vi "OnFrameAvailable_Event_Callback.vi"(4 "User Parameter":T1, 5 "Event Data":cluster{"sender":refnum<k24>, "e":refnum<k24>}, 6 "Control Ref":refnum<k24>, 7 "Event Common Data":T2) -> ()   [LabVIEW 2018]
uses:
  C:/Program Files/Spiricon/BeamSquared/M2.Automation.dll
  M2.Automation.dll
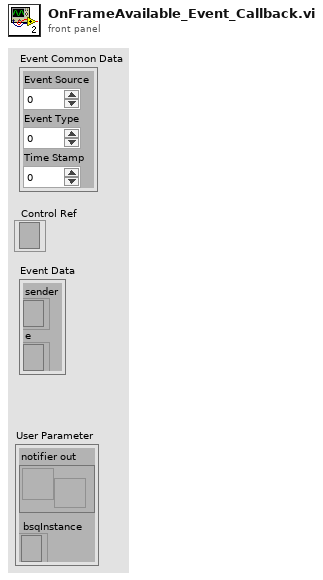
[diagram p1: front panel]
types:
  T1 = cluster{"notifier out":refnum<notifier>, "bsqInstance":refnum<k24>}
  T2 = cluster{"Event Source":i32, "Event Type":u32, "Time Stamp":u32}
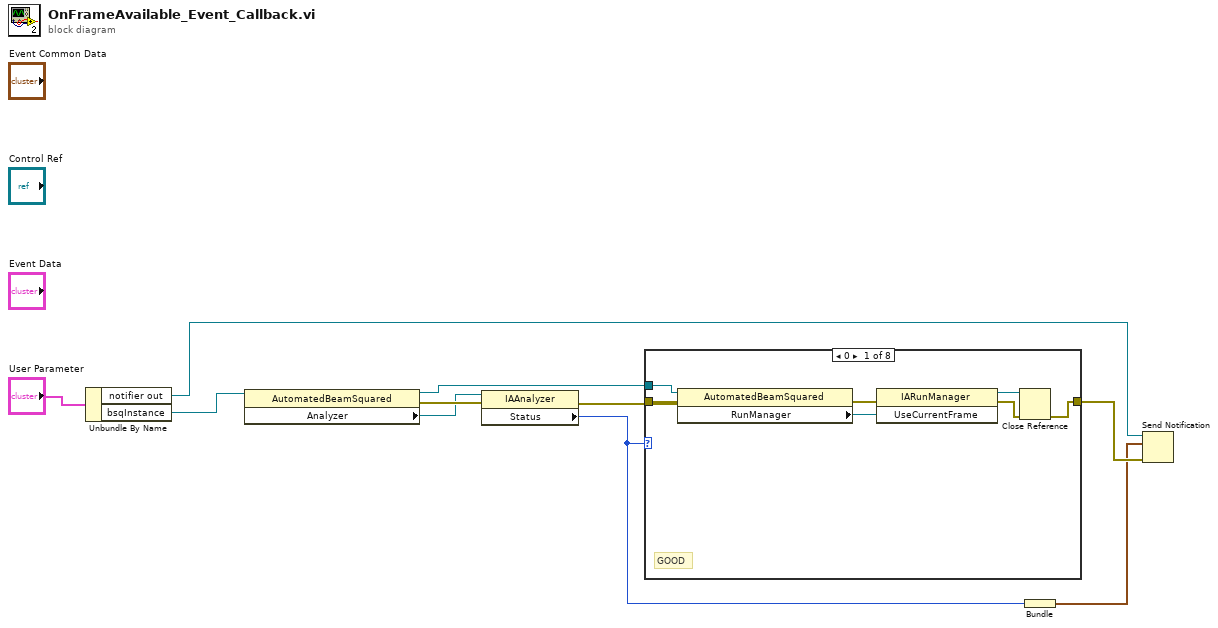
[diagram p0: block diagram]
diagram:
  n1 = Unbundle By Name("User Parameter") -> ("notifier out"=w9:refnum<notifier>, "bsqInstance"=w2:refnum<k24>)
  n2 = property class="AutomatedBeamSquared"(reference=w2) -> (reference out=w1:refnum<k24>, error out=w8:errorcluster, "Analyzer"=w7:refnum<k24>)  [unwired: 1 in]
  n3 = property class="IAAnalyzer"(reference=w7, error in=w8) -> (error out=w6:errorcluster, "Status"=w3:i32)  [unwired: 1 out]
  n4 = case shown="0" w3 {
    tunnel: w6 -> [w17 w18 w19 w20 w21 w22 w23 w24]
    tunnel: [w13 w18 w19 w20 w21 w22 w23 w24] -> w5
    tunnel: w1 -> [w11 _ _ _ _ _ _ _]
    frame 0 {
      # "GOOD"
      n5 = property class="AutomatedBeamSquared"(reference=w11, error in=w17) -> (error out=w16:errorcluster, "RunManager"=w15:refnum<k24>)  [unwired: 1 out]
      n6 = invoke class="IARunManager" method="UseCurrentFrame"(reference=w15, error in=w16) -> (reference out=w14:refnum<k24>, error out=w12:errorcluster)  [unwired: 1 in, 1 out]
      n7 = Close Reference(reference=w14, error in (no error)=w12) -> (error out=w13:errorcluster)
    }
    frame 1, Default {
      # "UNKNOWN"
    }
    frame 2 {
      # "BRIGHT"
    }
    frame 3 {
      # "DIM"
    }
    frame 4 {
      # "BIG"
    }
    frame 5 {
      # "ALIGNMENT"
    }
    frame 6 {
      # "SMALL"
    }
    frame 7 {
      # "NOT_ULTRACALED"
    }
  }
  n8 = Bundle("Status"=w3) -> (w4:cluster{"Status":i32})  [unwired: 1 in]
  n9 = Send Notification(notification=w4, notifier=w9, error in (no error)=w5) -> ()  [unwired: 2 out]
